vi "Measured Data Example (A).vi"() -> ()   [LabVIEW 2011]
uses:
  C:/Program Files/Metrohm Autolab/Autolab SDK 1.10/EcoChemie.Autolab.Sdk.dll
  EcoChemie.Autolab.Sdk.dll
panel:
  out "Numeric":i32
  out "GetSetDoubleValue":dbl
  in  "Signal Y":string(combo)
  in  "Signal X":string(combo)
  in  "ProcedureCommandList":string(combo)
  out "XY Graph":cluster{"Values":dbl[], "Values":dbl[]}(graph)
  out "Value Y":dbl[](array[numeric])
  out "Value X":dbl[](array[numeric])
  out "error out":errorcluster
  in  "Stop":bool
  in  "Procedure":path=path "Standard Nova Procedures/Cyclic voltammetry.nox"
  in  "Load":bool
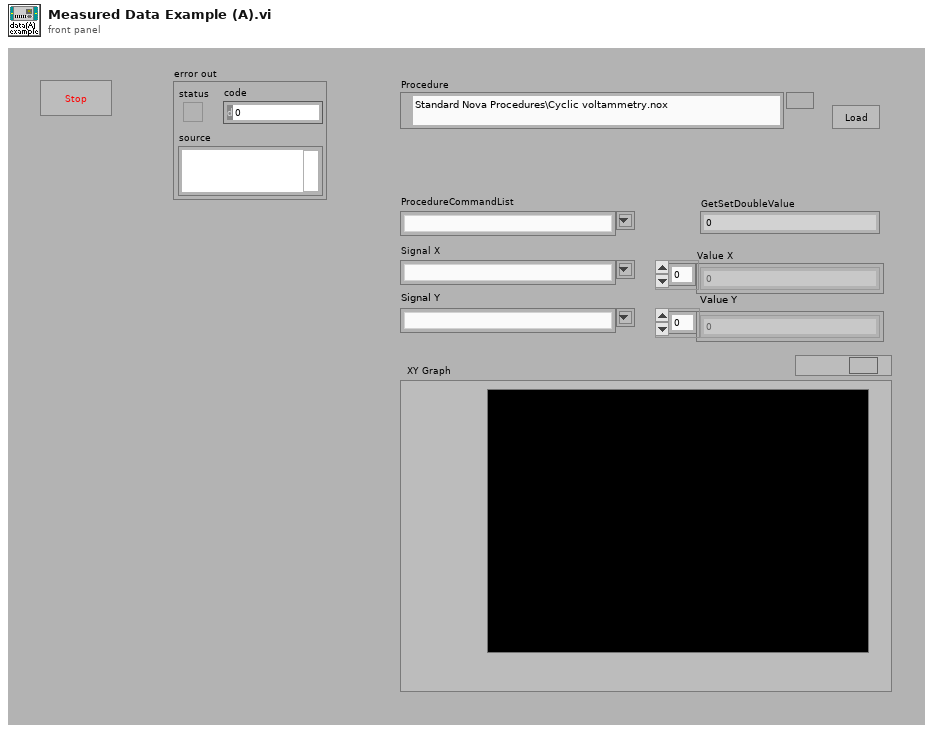
[diagram p1: front panel]
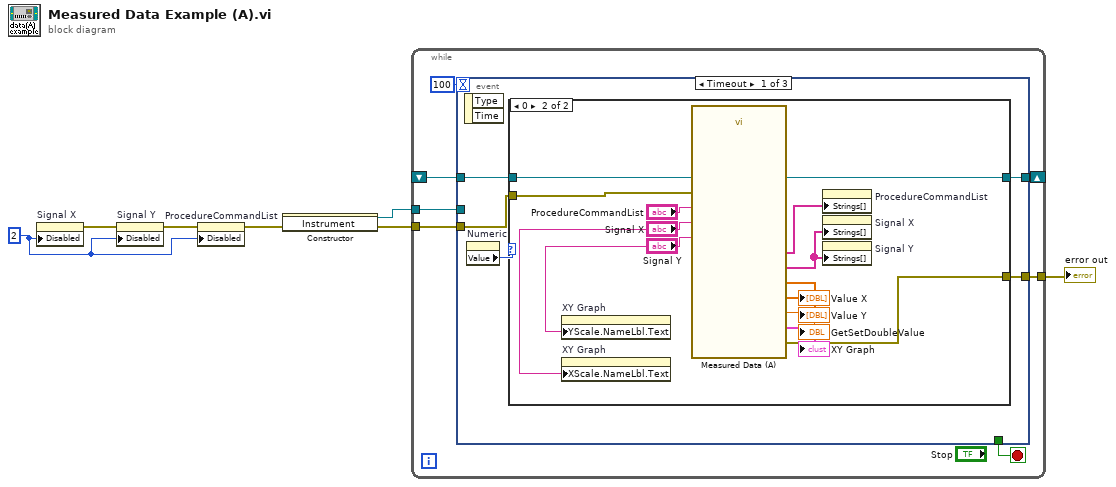
[diagram p0: block diagram]
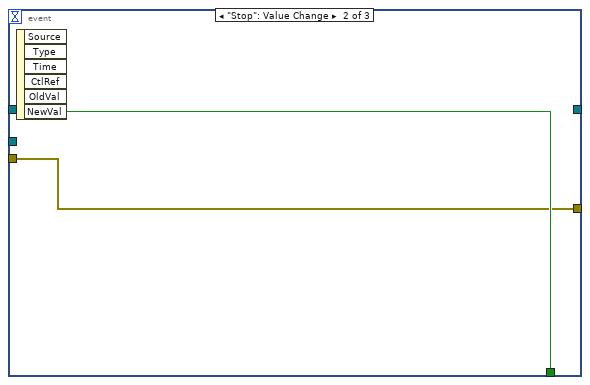
[diagram p3: hidden frame]
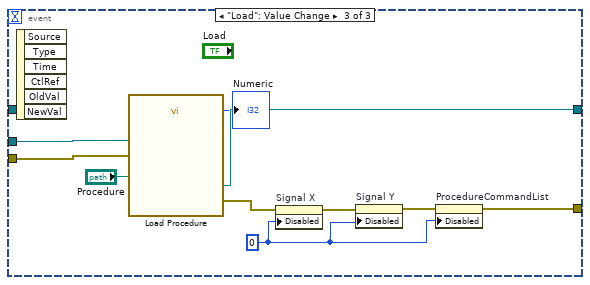
[diagram p4: hidden frame]
diagram:
  w5 = u8 2 ("Disabled")
  n1 = property on="Signal X" class="CmbBox"("Disabled"=w5) -> (error out=w7:errorcluster)  [unwired: 2 in, 1 out]
  n2 = property on="Signal Y" class="CmbBox"(error in=w7, "Disabled"=w5) -> (error out=w6:errorcluster)  [unwired: 1 in, 1 out]
  n3 = property on="ProcedureCommandList" class="CmbBox"(error in=w6, "Disabled"=w5) -> (error out=w3:errorcluster)  [unwired: 1 in, 1 out]
  n4 = constructor class="Instrument"(error in=w3) -> (reference out=w1:refnum<k24>, error out=w2:errorcluster)  [unwired: 2 in, 1 out]
  n5 = while {
    tunnel: w1 -> [w12]
    tunnel: [w11] -> w4
    tunnel: w2 -> [w10]
    shift-right: [w9] -> _
    shift-left: _ -> [w8]
    stop <- w13 stop-if-true
    n6 = event shown="[0] Timeout" {
      selector: _ -> [_ _ _]
      dyn-events: _ -> [_ _ _]
      timeout: 100 -> [_ _ _]
      tunnel: [_ w33 _] -> w13
      tunnel: w12 -> [_ _ w38]
      tunnel: [w16 w32 w37] -> w11
      tunnel: w10 -> [w18 w32 w36]
      tunnel: [w15 _ w35] -> w9
      tunnel: w8 -> [w15 _ _]
      event Timeout {
        n7 = event-data() -> ()  [unwired: 1 in, 2 out]
        n8 = property on="Numeric" class="DigNum (strict)"() -> ("Value"=w17:i32)  [unwired: 2 in, 2 out]
        n9 = case shown="0" w17 {
          tunnel: w18 -> [w19 w22]
          tunnel: w15 -> [_ w21]
          tunnel: [w19 w20] -> w16
          tunnel: w15 -> [_ _]
          frame 2, Default {
          }
          frame 0 {
            n10 = property on="XY Graph" class="XYGraph (strict)"("YScale.NameLbl.Text"="Signal Y") -> ()  [unwired: 2 in, 2 out]
            n11 = property on="XY Graph" class="XYGraph (strict)"("XScale.NameLbl.Text"="Signal X") -> ()  [unwired: 2 in, 2 out]
            n12 = call "Measured Data (A).vi"("LoadProcedure"=w21, "ProcedureCommandList"="ProcedureCommandList", "Signal X sel"="Signal X", "Signal Y sel"="Signal Y", "error in (no error)"=w22) -> ("Value Y"=→"Value Y":dbl[], "Signal Names"=w25:string[], "ProcedureCommandList"=w23:string[], "Value"=→"GetSetDoubleValue":dbl, "Value X"=→"Value X":dbl[], "XY Graph"=→"XY Graph":cluster{"Values":dbl[], "Values":dbl[]}, "error out"=w20:errorcluster)  [unwired: 4 in]
            n13 = property on="ProcedureCommandList" class="CmbBox"("Strings[]"=w23) -> ()  [unwired: 2 in, 2 out]
            n14 = property on="Signal X" class="CmbBox"("Strings[]"=w25) -> ()  [unwired: 2 in, 2 out]
            n15 = property on="Signal Y" class="CmbBox"("Strings[]"=w25) -> ()  [unwired: 2 in, 2 out]
          }
        }
      }
      event "Stop": Value Change {
        n16 = event-data() -> ("NewVal"=w33:bool)  [unwired: 1 in, 5 out]
      }
      event "Load": Value Change {
        w39 = u8 0 ("Disabled")
        n17 = event-data() -> ()  [unwired: 1 in, 6 out]
        n18 = call "Load Procedure.vi"("error in (no error)"=w36, "Procedure"="Procedure", "Instrument"=w38) -> ("error out"=w42:errorcluster, "Numeric"=→"Numeric":i32, "LoadProcedure"=w35:refnum<k24>)  [unwired: 5 in, 1 out]
        n19 = property on="Signal X" class="CmbBox"(error in=w42, "Disabled"=w39) -> (error out=w41:errorcluster)  [unwired: 1 in, 1 out]
        n20 = property on="Signal Y" class="CmbBox"(error in=w41, "Disabled"=w39) -> (error out=w40:errorcluster)  [unwired: 1 in, 1 out]
        n21 = property on="ProcedureCommandList" class="CmbBox"(error in=w40, "Disabled"=w39) -> (error out=w37:errorcluster)  [unwired: 1 in, 1 out]
      }
    }
  }
  "error out" <- w4
